vi "VibratomeGUI.vi"(8 "Error Out":errorcluster, 11 "Remote?":bool) -> ()   [LabVIEW 2018]
uses:
  Hardware Mfg/Thorlabs Translation Stages/Controls/Translation Stage Cluster.ctl
  Controls/Translation Stage Types.ctl
  Controls/Translation Stage Quick Status.ctl
  Controls/Translation Stage Quick Controls.ctl
  Controls/QueueNames.ctl
  Controls/Queue Manager Actions.ctl
  Controls/MessagePacket.ctl
  <vilib>/Utility/miscctls.llb/LVPointTypeDef.ctl
  Hardware Mfg/Thorlabs Translation Stages/Controls/Motion Translation Module Control.ctl
  Controls/Set Get Controls.ctl
  Controls/FGV Actions.ctl
panel:
  in  "Z STEP MOTION":enum16{"Fine", "Course", "Extra Course"}(ring)
  in  "Stop Button":bool
  in  "Slice":bool
  in  "Vibratome Controls":T1
  out "Message":string
  in  "Z Ctrl":T2
  out "Z Status":T3
  in  "Y Ctrl":T2
  out "Y Status":T3
  in  "X Ctrl":T2
  out "X Status":T3
  in  "XY STEP MOTION":enum16{"Fine", "Course", "Extra Course"}(ring)
  out "Cluster":cluster{"X":T4, "Y":T4, "Z":T4}
  in  "Exit":bool
  out "Processor Error Out":errorcluster
  out "GUI Error Out":errorcluster
  # "Vibratome Controls"
  # "Z Axis"
  # "Y Axis"
  # "X Axis"
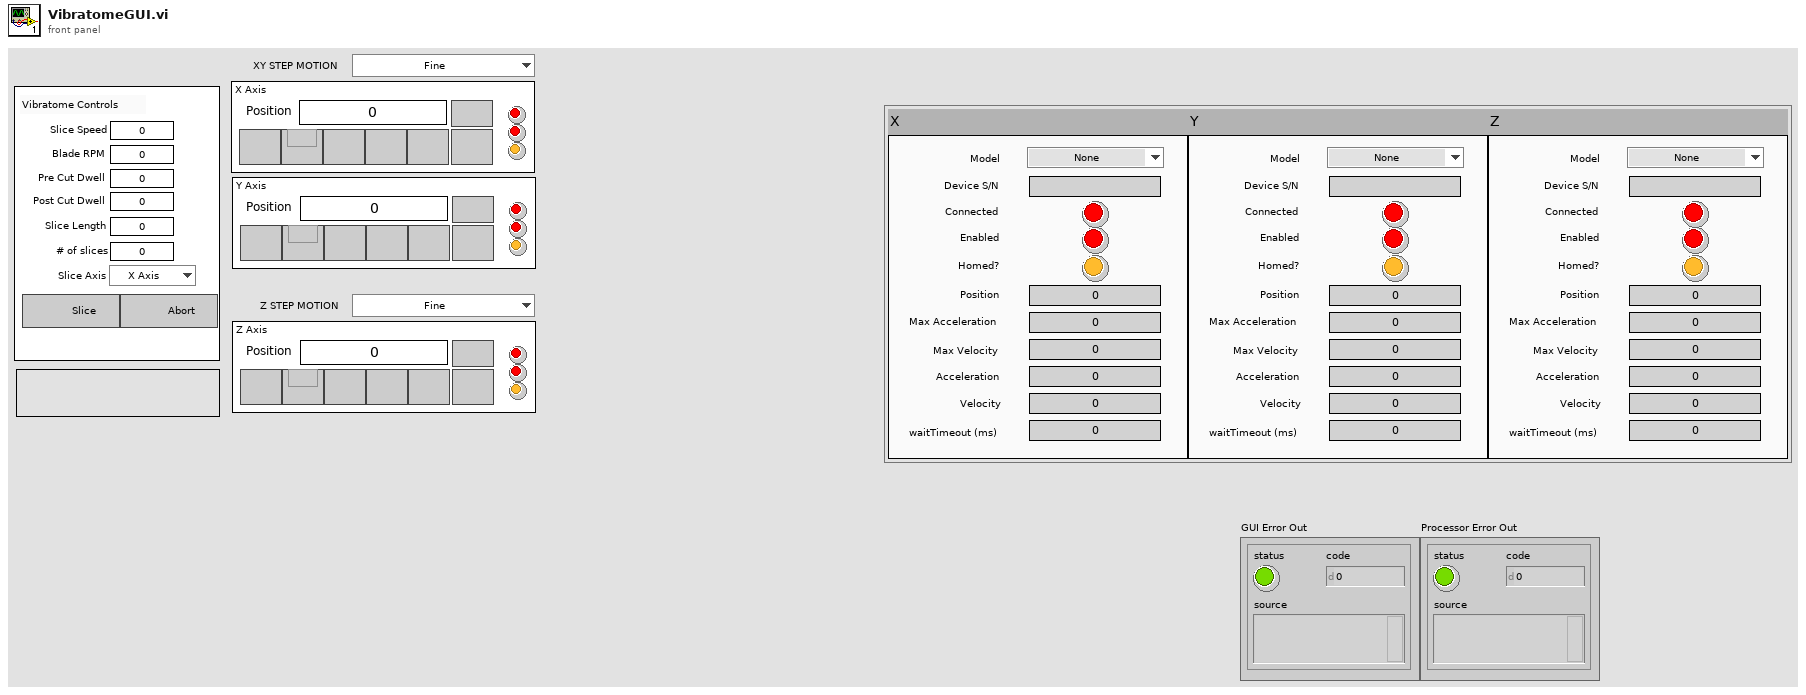
[diagram p1: front panel]
types:
  T1 = cluster{"Pre Cut Dwell":dbl, "Blade RPM":u16, "Slice Speed":dbl, "Post Cut Dwell":dbl, "Slice Length":dbl, "# of slices":dbl, "Slice Axis":enum16{"X Axis", "Y Axis", "Z Axis"}}
  T2 = typedef "Translation Stage Quick Controls.ctl" = cluster{"Position":dbl, "Next Button":bool, "Last Button":bool, "Previous Button":bool, "First Button":bool, "Home Button":bool, "Go":bool, "Settings Button":bool}
  T3 = typedef "Translation Stage Quick Status.ctl" = cluster{"Is.Enabled?":bool, "Is.Connected?":bool, "Is.Homed?":bool}
  T4 = typedef "Translation Stage Cluster.ctl" = cluster{"Position":dbl, "Is.Enabled?":bool, "Is.Connected?":bool, "Device SN":string, "AccelerationMaximum":dbl, "VelocityMaximum":dbl, "Acceleration":dbl, "Velocity":dbl, "waitTimeout (ms)":i32, "Model":T5, "Is.Homed?":bool}
  T5 = typedef "Translation Stage Types.ctl" = enum16{"None", "Thorlabs LTS", "Thorlabs MLJ"}
  T6 = typedef "MessagePacket.ctl" = cluster{"Message":string, "Parameter":variant}
  T7 = typedef "Queue Manager Actions.ctl" = enum16{"Init", "Enqueue", "Enqueue All", "Preview Queue", "Dequeue", "Get Status", "Flush Queue", "Flush All Queues", "Release All Queues", "Release Queue", "Enqueue at Opposite End"}
  T8 = typedef "QueueNames.ctl" = enum16{"Main GUI", "Main Scan Processor", "Main Processing", "Main Saving", "Main Display", "Main Table Stage GUI", "Main Table Stage Proc.", "Scan Engine", "Vibratome GUI", "Vibratome Processor", "Slice Engine"}
  T9 = enum32{"Invalid", "Default", "Floating", "Floating/Auto-Hide", "Modal"}
  T10 = enum32{"Invalid", "Standard", "Closed", "Hidden", "Minimized", "Maximized"}
  T11 = typedef "LVPointTypeDef.ctl" = cluster{"Horizontal":i16, "Vertical":i16}
  T12 = enum16{"Set Configuration", "Get Configuration", "Enable Motor", "Disable Motor", "Get Status", "Open Session", "Close Session", "Set Limits", "Get Limits"}
  T13 = typedef "FGV Actions.ctl" = enum16{"Init", "Set", "Get", "Clear"}
  T14 = typedef "Set Get Controls.ctl" = enum16{"Set", "Get"}
  T15 = typedef "Motion Translation Module Control.ctl" = enum16{"Init", "Home", "Status", "Velocity/Accel", "Position", "Jog", "Stop", "Uninit", "Enable", "Disable"}
  T16 = typedef "Translation Stage Parameters.ctl" = cluster{"X Stage":T4, "Y Stage":T4, "Z Stage":T4}
  T17 = typedef "System Parameters.ctl" = cluster{"Optical Parameters":T18, "Vibratome":T19, "Table Stages":T16, "Imaging Parameter":T20, "Galvo HW Parameters":cluster{"Analog Out Channel":tag, "Min Voltage":dbl, "Max Voltage":dbl, "Pixel Clock Source":tag, "Sample Rate":dbl, "Line Clock Out Ch":tag}, "Alazar parameters":T22, "Mosaic Paramter":cluster{"X Axis":cluster{"Start [mm]":dbl, "Steps [pts]":dbl, "End [mm]":dbl}, "Y Axis":cluster{"Start [mm]":dbl, "Steps [pts]":dbl, "End [mm]":dbl}, "Scan Pattern":enum16{"Uni-directional", "Bi-Directional", "Spiral Out", "Spiral In"}, "Overlap Options":cluster{"Overlap Type":enum16{"No Overlap", "X Only", "Y Only", "X and Y"}, "Percent Overlap":u8, "Justify":enum16{"Start", "Center", "End"}}}, "Manual Controls":T29, "Vibratome Axis":T32}
  T18 = typedef "Optical Parameters.ctl" = cluster{"Obj. Focal Length [mm]":dbl, "Scan Lens EFL[mm]":dbl, "Tube Lens EFL[mm]":dbl, "Galvo V Range (+/-)":dbl, "Galvo Max Half Angle [Deg]":dbl, "Max Galvo Range[%]":dbl}
  T19 = typedef "Vibratome Parameters.ctl" = cluster{"Z Bottom [mm]":dbl, "Pre Cut Dwell [s]":dbl, "Blade Frequency [RPM]":u16, "Slice Speed [mm/s]":dbl, "Post Cut Dwell [s]":dbl, "Ramp Time [s]":dbl, "Start X [mm]":dbl, "Start Y [mm]":dbl, "Slice Length [mm]":dbl, "Slice Axis":enum16{"X Axis", "Y Axis", "Z Axis"}, "Controller VISA Ref":refnum<visa-resource-name>}
  T20 = typedef "Imaging Parameters.ctl" = cluster{"Raster Scan Direction":T21, "Pixel Dwell Time [Clock Cycles]":u16, "Flyback Time [Clock Cycles]":u16, "XY Center [um]":cluster{"X":dbl, "Y":dbl}, "Pixel Step Size [um]":dbl, "XY Image Size":enum16{"32 x 32", "64 x 64", "128 x 128", "256 x 256", "512 x 512", "1024 x 1024", "2048 x 2048"}, "Custom":bool, "Custom Size":cluster{"X":u16, "Y":u16}, "Line Averages":u8}
  T21 = typedef "Scan Direction.ctl" = enum16{"Uni Directional", "Bi Directional", "None"}
  T22 = typedef "Alazar parameters.ctl" = cluster{"Trigger Settings":cluster{"General Trigger Settings":T23, "Trigger Engine 1":T24, "Trigger Engine 2":T24}, "Device ID":T25, "Ch A Input Control":T26, "Ch B Input Control":T26, "Acq Settings":T27, "Capture Clock":T28}
  T23 = typedef "General Trigger Settings.ctl" = cluster{"Trigger Operation":u32, "Coupling ID":u32, "Range ID":u32, "Delay":u32, "Timeout Ticks":u32, "Mode":u32, "Parameter":u32}
  T24 = typedef "Trigger Engine Controls.ctl" = cluster{"Trigger Engine":u32, "Source":u32, "Slope":u32, "Level":u32}
  T25 = typedef "Alazar Device ID.ctl" = cluster{"System ID":u32, "Board ID":u32}
  T26 = typedef "Channel Input Controls.ctl" = cluster{"Channel":u8, "Coupling":u32, "Range":u32, "Impedance":u32}
  T27 = typedef "Alazar Acquisition Settings.ctl" = cluster{"Record Length":u32, "Offset":u32, "Records Per Buffer":u32, "Records Count (Records/Acq)":u32, "Window Type":u32, "Footer":u32, "Samples per record":u32, "Output Format":u32}
  T28 = typedef "Clock Controls.ctl" = cluster{"Sample Rate":u32, "Decimation":u32, "Source":u32, "Edge":u32}
  T29 = typedef "Manual Controls.ctl" = cluster{"Z0":dbl, "Z0 image":dbl, "stripped path":path, "Save parameters":T30, "Center Galvos":bool, "Acquisition mode":T31, "PSOCT Channel":u32, "Save":bool, "AIP rotation angle":dbl, "Scan Parameters":cluster{"# Scan":cluster{"#Ascan":i32, "#Bscan":i32}, "# Rpt":cluster{"#ARpt":i32, "#BRpt":i32}, "Aline Rate":u16, "# Extra":cluster{"# ARpt_extra":i32, "#Brtn_extra":i32}}, "ROI Parameters":cluster{"ROI (mm)":cluster{"X (mm)":dbl, "Y (mm)":dbl}, "Shift (mm)":cluster{"Xshift (mm)":sgl, "Yshift (mm)":sgl}}, "Objective":u16}
  T30 = typedef "FFT parameters.ctl" = cluster{"start pixel":i32, "#pixels to save":i32}
  T31 = typedef "FFT mode.ctl" = enum16{"ThorOCT B line", "ThorOCT Spectral", "ThorOCT FFT", "Alazar B line", "Alazar FFT", "GPU FFT", "Alazar Spectral"}
  T32 = typedef "Vibratome Param.ctl" = cluster{"Start [mm](Next cut height)":dbl, "thick slice[um]":dbl, "#repitition":u16, "thin slice[um]":dbl, "#thin slices":u16}
  T33 = cluster{"Z Bottom [mm]":dbl, "Pre Cut Dwell [s]":dbl, "Blade Frequency [RPM]":u16, "Slice Speed [mm/s]":dbl, "Post Cut Dwell [s]":dbl, "Ramp Time [s]":dbl, "Start X [mm]":dbl, "Start Y [mm]":dbl, "Slice Length [mm]":dbl, "Slice Axis":enum16{"X Axis", "Y Axis", "Z Axis"}, "Controller VISA Ref":refnum<visa-resource-name>}
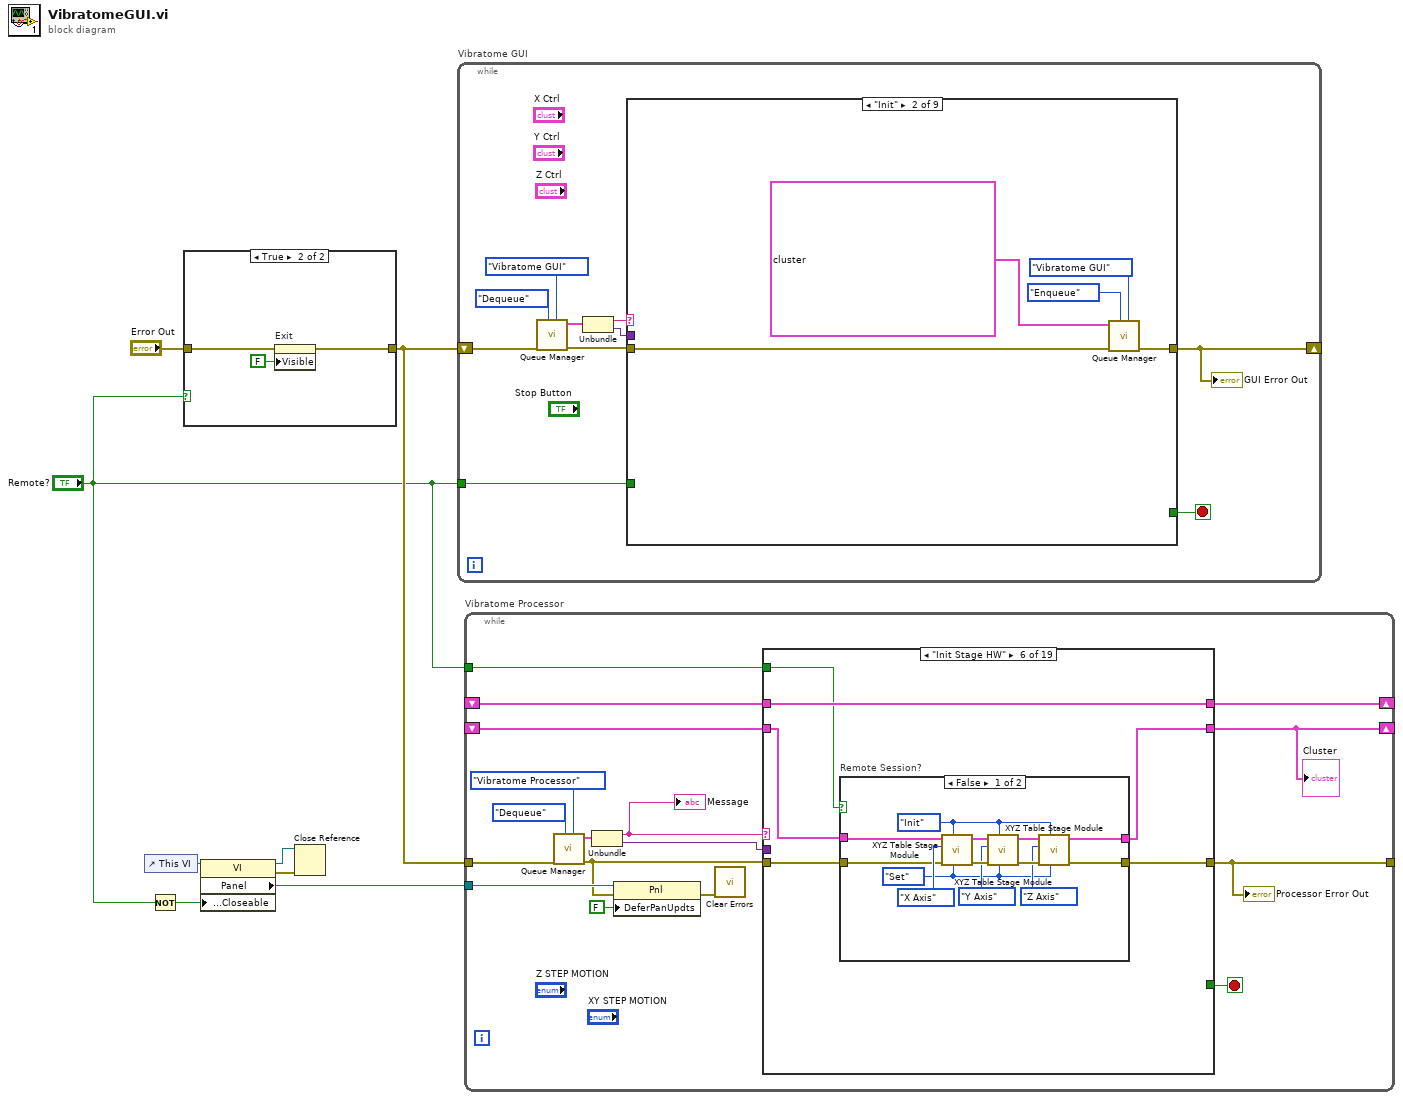
[diagram p0: block diagram]
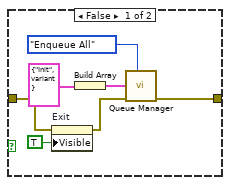
[diagram p2: hidden frame]
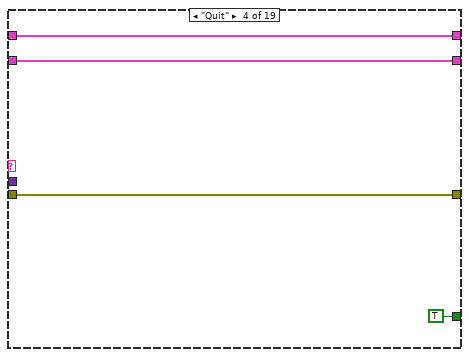
[diagram p6: hidden frame]
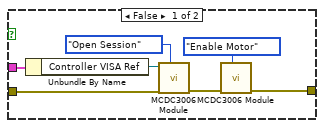
[diagram p10: hidden frame]
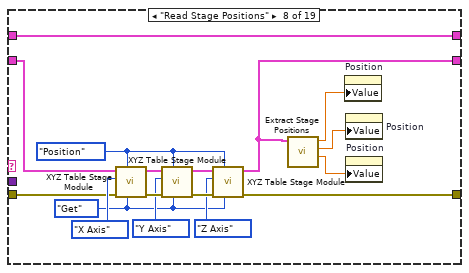
[diagram p11: hidden frame]
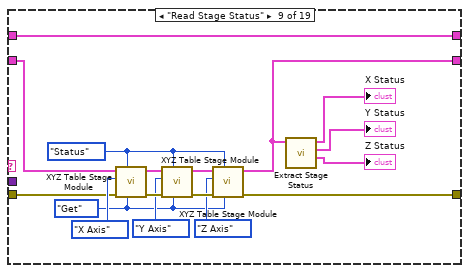
[diagram p12: hidden frame]
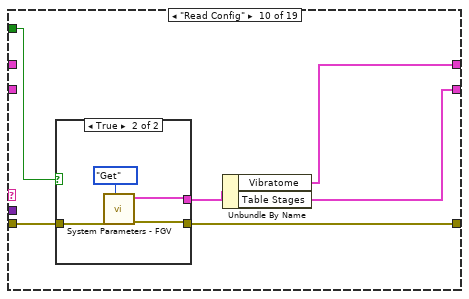
[diagram p13: hidden frame]
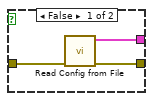
[diagram p14: hidden frame]
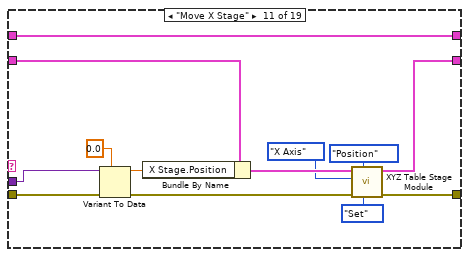
[diagram p15: hidden frame]
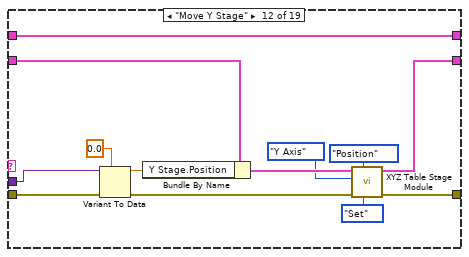
[diagram p16: hidden frame]
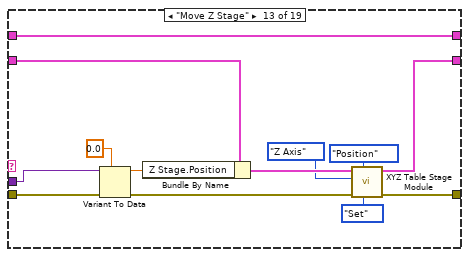
[diagram p17: hidden frame]
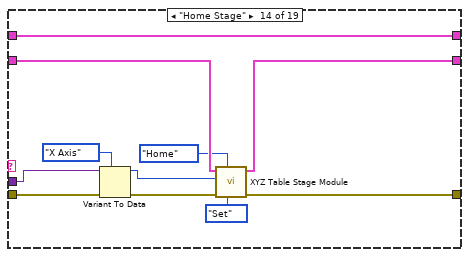
[diagram p18: hidden frame]
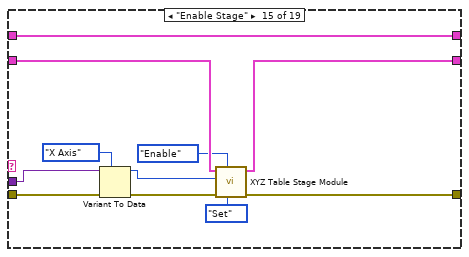
[diagram p19: hidden frame]
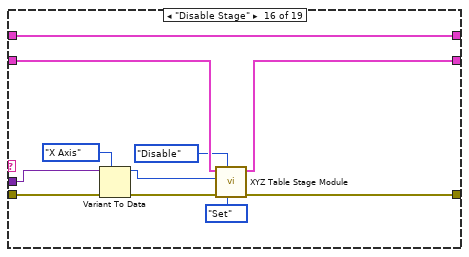
[diagram p20: hidden frame]
diagram:
  n1 = control-ref of="This VI"() -> (w7:refnum<vi>)
  n2 = Not(x="Remote?") -> (.not. x?=w1:bool)
  n3 = case shown="True" "Remote?" {
    tunnel: [w12 w17] -> w8
    tunnel: "Error Out" -> [w10 w18]
    frame False {
      n4 = property on="Exit" class="Bool"(error in=w10, "Visible"=TRUE) -> (error out=w9:errorcluster)  [unwired: 1 in, 1 out]
      n5 = Build Array(T6 {"Message"="Init", "Parameter"=variant} ("Message Packet [In]")) -> (w13:T6[])
      n6 = call "Queue Manager.vi"("Action"=Queue_Manager_Actions."Enqueue All", "Error In"=w9, "Message Packet Array"=w13) -> ("Error Out"=w12:errorcluster)  [unwired: 4 in, 4 out]
    }
    frame True {
      n7 = property on="Exit" class="Bool"(error in=w18, "Visible"=FALSE) -> (error out=w17:errorcluster)  [unwired: 1 in, 1 out]
    }
  }
  n8 = property class="VI"(reference=w7, "Front Panel.Closeable"=w1) -> (reference out=w5:refnum<vi>, error out=w6:errorcluster, "Panel"=w4:refnum<vi>)  [unwired: 1 in]
  n9 = Close Reference(reference=w5, error in (no error)=w6) -> ()  [unwired: 1 out]
  n10 = while "Vibratome GUI" {
    shift-right: [w28] -> _
    shift-left: w8 -> [w26]
    tunnel: "Remote?" -> [w19]
    stop <- w21 stop-if-true
    n11 = call "Queue Manager.vi"("Queue Name"=QueueNames."Vibratome GUI", "Action"=Queue_Manager_Actions."Dequeue", "Error In"=w26) -> ("Error Out"=w25:errorcluster, "Message Packet [Out]"=w24:T6)  [unwired: 4 in, 3 out]
    n12 = Unbundle(w24) -> ("Message"=w23:string, "Parameter"=w22:variant)
    n13 = case shown="\"Init\"" w23 {
      tunnel: w25 -> [w29 w30 w35 w36 w38 w42 w45 w118 w130]
      tunnel: [w29 w31 w35 w36 w37 w42 w44 w119 w130] -> w28
      tunnel: w22 -> [_ _ _ _ _ _ _ _ _]
      tunnel: [_ _ _ _ _ _ _ _ TRUE] -> w21
      tunnel: w19 -> [_ _ _ _ _ _ w43 w113 _]
      frame "Unknown", Default {
      }
      frame "Init" {
        n14 = call "Queue Manager.vi"("Queue Name"=QueueNames."Vibratome GUI", "Action"=Queue_Manager_Actions."Enqueue", "Error In"=w30, "Message Packet Array"=T6[] [{"Message"="Init Variables", "Parameter"=variant}, {"Message"="Set Front Panel", "Parameter"=variant}, {"Message"="Load User Settings", "Parameter"=variant}, {"Message"="Configure Hardware", "Parameter"=variant}, {"Message"="Wait for Complete", "Parameter"=variant}, {"Message"="Wait for User Input", "Parameter"=variant}]) -> ("Error Out"=w31:errorcluster)  [unwired: 3 in, 4 out]
      }
      frame "Init Variables" {
      }
      frame "Load User Settings" {
      }
      frame "Configure Hardware" {
        n15 = call "Queue Manager.vi"("Queue Name"=QueueNames."Vibratome Processor", "Action"=Queue_Manager_Actions."Enqueue", "Error In"=w38, "Message Packet Array"=T6[] [{"Message"="Read Config", "Parameter"=variant}, {"Message"="Init Stage HW", "Parameter"=variant}, {"Message"="Read Stage Status", "Parameter"=variant}, {"Message"="Read Stage Positions", "Parameter"=variant}, {"Message"="Init Vibratome HW", "Parameter"=variant}, {"Message"="Finished Init", "Parameter"=variant}]) -> ("Error Out"=w37:errorcluster)  [unwired: 3 in, 4 out]
      }
      frame "Wait for Complete" {
      }
      frame "Wait for User Input" {
        n16 = event shown="[1] Panel Close;  Application Instance Close;  \"Exit\": Value Change" {
          selector: _ -> [_ _ _ _ _ _]
          dyn-events: _ -> [_ _ _ _ _ _]
          timeout: _ -> [_ _ _ _ _ _]
          tunnel: w45 -> [w46 w49 w57 w79 w94 w109]
          tunnel: [w46 w48 w62 w66 w81 w96] -> w44
          tunnel: w43 -> [_ w47 _ _ _ _]
          event Timeout {
            n17 = event-data() -> ()  [unwired: 1 in, 3 out]
          }
          event Panel Close; Application Instance Close; "Exit": Value Change {
            n18 = event-data() -> ()  [unwired: 1 in, 3 out]
            n19 = case shown="True" w47 {
              tunnel: w49 -> [w53 w55]
              tunnel: [w52 w55] -> w48
              frame False {
                n20 = Build Array(T6 {"Message"="Exit", "Parameter"=variant} ("Message Packet [In]")) -> (w50:T6[])
                n21 = call "Queue Manager.vi"("Action"=Queue_Manager_Actions."Enqueue All", "Error In"=w53, "Message Packet Array"=w50) -> ("Error Out"=w52:errorcluster)  [unwired: 4 in, 4 out]
              }
              frame True {
              }
            }
          }
          event "Slice": Value Change {
            n22 = event-data() -> ()  [unwired: 1 in, 6 out]
            n23 = Build Array(T6 {"Message"="Wait for User Input", "Parameter"=variant} ("Message Packet [In]")) -> (w60:T6[])
            n24 = call "Queue Manager.vi"("Queue Name"=QueueNames."Vibratome GUI", "Action"=Queue_Manager_Actions."Enqueue", "Error In"=w57, "Message Packet Array"=w60) -> ("Error Out"=w62:errorcluster)  [unwired: 3 in, 4 out]
            n25 = call "Queue Manager.vi"("Queue Name"=QueueNames."Vibratome Processor", "Action"=Queue_Manager_Actions."Enqueue", "Error In"=w57, "Message Packet Array"=T6[] [{"Message"="Slice", "Parameter"=variant}, {"Message"="Finished", "Parameter"=variant}]) -> ()  [unwired: 3 in, 5 out]
          }
          event Value Change {
            n26 = event-data() -> ()  [unwired: 1 in, 1 out]
            n27 = property on="Position" class="DigNum (strict)"(error in=w79) -> (error out=w76:errorcluster, "Value"=w74:dbl)  [unwired: 1 in, 1 out]
            n28 = Bundle By Name(cluster=T6 {"Message"="Move X Stage", "Parameter"=variant} ("Message Packet [In]"), "Parameter"=w74) -> (w73:T6)
            n29 = Build Array(w73, T6 {"Message"="Finished", "Parameter"=variant} ("Message Packet [In]")) -> (w72:T6[])
            n30 = call "Queue Manager.vi"("Queue Name"=QueueNames."Vibratome Processor", "Action"=Queue_Manager_Actions."Enqueue", "Error In"=w76, "Message Packet Array"=w72) -> ("Error Out"=w67:errorcluster)  [unwired: 3 in, 4 out]
            n31 = Build Array(T6 {"Message"="Wait for User Input", "Parameter"=variant} ("Message Packet [In]")) -> (w68:T6[])
            n32 = call "Queue Manager.vi"("Queue Name"=QueueNames."Vibratome GUI", "Action"=Queue_Manager_Actions."Enqueue", "Error In"=w67, "Message Packet Array"=w68) -> ("Error Out"=w66:errorcluster)  [unwired: 3 in, 4 out]
          }
          event Value Change {
            n33 = event-data() -> ()  [unwired: 1 in, 1 out]
            n34 = property on="Position" class="DigNum (strict)"(error in=w94) -> (error out=w91:errorcluster, "Value"=w89:dbl)  [unwired: 1 in, 1 out]
            n35 = Bundle By Name(cluster=T6 {"Message"="Move Y Stage", "Parameter"=variant} ("Message Packet [In]"), "Parameter"=w89) -> (w88:T6)
            n36 = Build Array(w88, T6 {"Message"="Finished", "Parameter"=variant} ("Message Packet [In]")) -> (w87:T6[])
            n37 = call "Queue Manager.vi"("Queue Name"=QueueNames."Vibratome Processor", "Action"=Queue_Manager_Actions."Enqueue", "Error In"=w91, "Message Packet Array"=w87) -> ("Error Out"=w82:errorcluster)  [unwired: 3 in, 4 out]
            n38 = Build Array(T6 {"Message"="Wait for User Input", "Parameter"=variant} ("Message Packet [In]")) -> (w83:T6[])
            n39 = call "Queue Manager.vi"("Queue Name"=QueueNames."Vibratome GUI", "Action"=Queue_Manager_Actions."Enqueue", "Error In"=w82, "Message Packet Array"=w83) -> ("Error Out"=w81:errorcluster)  [unwired: 3 in, 4 out]
          }
          event Value Change {
            n40 = event-data() -> ()  [unwired: 1 in, 1 out]
            n41 = property on="Position" class="DigNum (strict)"(error in=w109) -> (error out=w106:errorcluster, "Value"=w104:dbl)  [unwired: 1 in, 1 out]
            n42 = Bundle By Name(cluster=T6 {"Message"="Move Z Stage", "Parameter"=variant} ("Message Packet [In]"), "Parameter"=w104) -> (w103:T6)
            n43 = Build Array(w103, T6 {"Message"="Finished", "Parameter"=variant} ("Message Packet [In]")) -> (w102:T6[])
            n44 = call "Queue Manager.vi"("Queue Name"=QueueNames."Vibratome Processor", "Action"=Queue_Manager_Actions."Enqueue", "Error In"=w106, "Message Packet Array"=w102) -> ("Error Out"=w97:errorcluster)  [unwired: 3 in, 4 out]
            n45 = Build Array(T6 {"Message"="Wait for User Input", "Parameter"=variant} ("Message Packet [In]")) -> (w98:T6[])
            n46 = call "Queue Manager.vi"("Queue Name"=QueueNames."Vibratome GUI", "Action"=Queue_Manager_Actions."Enqueue", "Error In"=w97, "Message Packet Array"=w98) -> ("Error Out"=w96:errorcluster)  [unwired: 3 in, 4 out]
          }
        }
      }
      frame "Set Front Panel" {
        n47 = Select(t=T10."Hidden" ("Front Panel Window:State"), s=w113, f=T10."Standard" ("Front Panel Window:State")) -> (s? t:f=w114:T10)
        n48 = control-ref of="This VI"() -> (w117:refnum<vi>)
        n49 = Select(t=T9."Default" ("Front Panel Window:Behavior"), s=w113, f=T9."Modal") -> (s? t:f=w110:T9)
        n50 = property class="VI"(reference=w117, error in=w118, "FP.State"=w114, "FP.Behavior"=w110) -> (error out=w121:errorcluster, "Panel"=w124:refnum<vi>)  [unwired: 1 out]
        n51 = property class="Pnl"(reference=w124, error in=w121) -> (error out=w122:errorcluster, "Panes[]"=w123:refnum<vi>[])  [unwired: 1 out]
        n52 = for {
          tunnel: w123 -> [w128] mode=indexing
          tunnel: w122 -> [w126]
          tunnel: [w125] -> w120 mode=indexing
          n53 = property class="Pane"(reference=w128, error in=w126, "Origin"=T11 {"Horizontal"=0, "Vertical"=0}) -> (error out=w125:errorcluster)  [unwired: 1 out]
        }
        n54 = Merge Errors(w120) -> (w119:errorcluster)
      }
      frame "Exit" {
      }
    }
    "GUI Error Out" <- w28
  }
  n55 = while "Vibratome Processor" {
    tunnel: w8 -> [w145]
    tunnel: [w147] -> _
    shift-right: [w136] -> _
    shift-left: _ -> [w139]
    shift-right: [w138] -> _
    shift-left: _ -> [w137]
    tunnel: w4 -> [w135]
    tunnel: "Remote?" -> [w131]
    stop <- w141 stop-if-true
    n56 = call "Queue Manager.vi"("Queue Name"=QueueNames."Vibratome Processor", "Action"=Queue_Manager_Actions."Dequeue", "Error In"=w145) -> ("Error Out"=w133:errorcluster, "Message Packet [Out]"=w144:T6)  [unwired: 4 in, 3 out]
    n57 = Unbundle(w144) -> ("Message"=w143:string, "Parameter"=w142:variant)
    "Message" <- w143
    n58 = property class="Pnl"(reference=w135, error in=w133, "DeferPanUpdts"=FALSE ("Defer Panel Updates")) -> (error out=w132:errorcluster)  [unwired: 1 out]
    n59 = call <vilib>:"Clear Errors.vi"("error in (no error)"=w132) -> ()  [unwired: 5 in, 2 out]
    n60 = case shown="\"Init Stage HW\"" w143 {
      tunnel: w133 -> [w150 w153 w154 w158 w161 w166 w186 w202 w219 w235 w255 w268 w281 w292 w303 w314 w319 w325 w345]
      tunnel: [w150 w153 w154 w158 w161 w167 w184 w210 w227 w233 w254 w267 w280 w291 w302 w313 w318 w324 w329] -> w147
      tunnel: w142 -> [_ _ _ _ _ _ _ _ _ _ w252 w265 w278 w289 w300 w311 _ _ _]
      tunnel: [_ _ _ TRUE _ _ _ _ _ _ _ _ _ _ _ _ _ _ _] -> w141
      tunnel: [w149 w152 w156 w160 _ w163 w187 w196 w217 w234 w251 w264 w277 w285 w296 w307 w316 w326 w338] -> w136
      tunnel: w139 -> [w149 w152 w156 w160 _ w165 w187 w201 w218 _ w247 w260 w273 w286 w297 w308 w316 w326 w341]
      tunnel: [w148 w151 w155 w159 _ w164 w185 w200 w213 w232 w243 w256 w269 w282 w293 w304 w320 w327 w332] -> w138
      tunnel: w137 -> [w148 w151 w155 w159 _ w164 w185 w200 w213 _ w243 w256 w269 w282 w293 w304 w320 w327 w332]
      tunnel: w131 -> [_ _ _ _ _ w162 w183 _ _ w230 _ _ _ _ _ _ _ _ _]
      frame "Unknown", Default {
      }
      frame "Finished Init" {
      }
      frame "Finished" {
      }
      frame "Quit" {
      }
      frame "Init" {
      }
      frame "Init Stage HW" {
        n61 = case "Remote Session?" shown="False" w162 {
          tunnel: [w178 w181] -> w167
          tunnel: w166 -> [w170 w181]
          tunnel: w165 -> [w169 w182]
          tunnel: [w168 w182] -> w163
          frame False {
            w171 = Set_Get_Controls."Set" ("Set/Get")
            w177 = Motion_Translation_Module_Control."Init" ("Action")
            n62 = call "XYZ Table Stage Module.vi"("Set/Get"=w171, "Action"=w177, "Error In"=w170, "Axis"=enum16{"X Axis", "Y Axis", "Z Axis"}."X Axis", "Table Stages"=w169) -> ("Error Out"=w180:errorcluster, "Table Stages [out]"=w176:T16)  [unwired: 5 in]
            n63 = call "XYZ Table Stage Module.vi"("Set/Get"=w171, "Action"=w177, "Error In"=w180, "Axis"=enum16{"X Axis", "Y Axis", "Z Axis"}."Y Axis", "Table Stages"=w176) -> ("Error Out"=w179:errorcluster, "Table Stages [out]"=w175:T16)  [unwired: 5 in]
            n64 = call "XYZ Table Stage Module.vi"("Set/Get"=w171, "Action"=w177, "Error In"=w179, "Axis"=enum16{"X Axis", "Y Axis", "Z Axis"}."Z Axis", "Table Stages"=w175) -> ("Error Out"=w178:errorcluster, "Table Stages [out]"=w168:T16)  [unwired: 5 in]
          }
          frame True {
          }
        }
      }
      frame "Init Vibratome HW" {
        n65 = case "Remote Session?" shown="True" w183 {
          tunnel: w186 -> [w193 w195]
          tunnel: w185 -> [w191 _]
          tunnel: [w189 w195] -> w184
          frame False {
            n66 = Unbundle By Name(w191) -> ("Controller VISA Ref"=w190:refnum<visa-resource-name>)
            n67 = call "MCDC3006 Module.vi"("Actions"=T12."Open Session", "Error In"=w193, "VISA resource name"=w190) -> ("Error Out"=w192:errorcluster)  [unwired: 4 in, 4 out]
            n68 = call "MCDC3006 Module.vi"("Actions"=T12."Enable Motor", "Error In"=w192) -> ("Error Out"=w189:errorcluster)  [unwired: 5 in, 4 out]
          }
          frame True {
          }
        }
      }
      frame "Read Stage Positions" {
        w203 = Set_Get_Controls."Get" ("Set/Get")
        w209 = Motion_Translation_Module_Control."Position" ("Action")
        n69 = call "XYZ Table Stage Module.vi"("Set/Get"=w203, "Action"=w209, "Error In"=w202, "Axis"=enum16{"X Axis", "Y Axis", "Z Axis"}."X Axis", "Table Stages"=w201) -> ("Error Out"=w212:errorcluster, "Table Stages [out]"=w208:T16)  [unwired: 5 in]
        n70 = call "XYZ Table Stage Module.vi"("Set/Get"=w203, "Action"=w209, "Error In"=w212, "Axis"=enum16{"X Axis", "Y Axis", "Z Axis"}."Y Axis", "Table Stages"=w208) -> ("Error Out"=w211:errorcluster, "Table Stages [out]"=w207:T16)  [unwired: 5 in]
        n71 = call "XYZ Table Stage Module.vi"("Set/Get"=w203, "Action"=w209, "Error In"=w211, "Axis"=enum16{"X Axis", "Y Axis", "Z Axis"}."Z Axis", "Table Stages"=w207) -> ("Error Out"=w210:errorcluster, "Table Stages [out]"=w196:T16)  [unwired: 5 in]
        n72 = call "Extract Stage Positions.vi"("Table Stages"=w196) -> ("Z Stage.Position"=w197:dbl, "Y Stage.Position"=w198:dbl, "X Stage.Position"=w199:dbl)  [unwired: 8 in]
        n73 = property on="Position" class="DigNum (strict)"("Value"=w199) -> ()  [unwired: 2 in, 2 out]
        n74 = property on="Position" class="DigNum (strict)"("Value"=w198) -> ()  [unwired: 2 in, 2 out]
        n75 = property on="Position" class="DigNum (strict)"("Value"=w197) -> ()  [unwired: 2 in, 2 out]
      }
      frame "Read Stage Status" {
        w220 = Set_Get_Controls."Get" ("Set/Get")
        w226 = Motion_Translation_Module_Control."Status" ("Action")
        n76 = call "XYZ Table Stage Module.vi"("Set/Get"=w220, "Action"=w226, "Error In"=w219, "Axis"=enum16{"X Axis", "Y Axis", "Z Axis"}."X Axis", "Table Stages"=w218) -> ("Error Out"=w229:errorcluster, "Table Stages [out]"=w225:T16)  [unwired: 5 in]
        n77 = call "XYZ Table Stage Module.vi"("Set/Get"=w220, "Action"=w226, "Error In"=w229, "Axis"=enum16{"X Axis", "Y Axis", "Z Axis"}."Y Axis", "Table Stages"=w225) -> ("Error Out"=w228:errorcluster, "Table Stages [out]"=w224:T16)  [unwired: 5 in]
        n78 = call "XYZ Table Stage Module.vi"("Set/Get"=w220, "Action"=w226, "Error In"=w228, "Axis"=enum16{"X Axis", "Y Axis", "Z Axis"}."Z Axis", "Table Stages"=w224) -> ("Error Out"=w227:errorcluster, "Table Stages [out]"=w217:T16)  [unwired: 5 in]
        n79 = call "Extract Stage Status.vi"("Table Stages"=w217) -> ("Z Stage"=→"Z Status":T3, "Y Stage"=→"Y Status":T3, "X Stage"=→"X Status":T3)  [unwired: 8 in]
      }
      frame "Read Config" {
        n80 = case shown="True" w230 {
          tunnel: w235 -> [w238 w241]
          tunnel: [w237 w240] -> w233
          tunnel: [w236 w239] -> w231
          frame False {
            n81 = call "Read Config from File.vi"("error in (no error)"=w238) -> ("error out"=w237:errorcluster, "System Parameters"=w236:T17)  [unwired: 9 in]
          }
          frame True {
            n82 = call "System Parameters - FGV.vi"("Actions"=FGV_Actions."Get", "Error In"=w241) -> ("Error Out"=w240:errorcluster, "System Parameters [Out]"=w239:T17)  [unwired: 8 in]
          }
        }
        n83 = Unbundle By Name(w231) -> ("Vibratome"=w232:T19, "Table Stages"=w234:T16)
      }
      frame "Move X Stage" {
        n84 = Variant To Data(error in=w255, type=0.0 ("Value"), Variant=w252) -> (data=w246:dbl, error out=w253:errorcluster)
        n85 = Bundle By Name(cluster=w247, "X Stage.Position"=w246) -> (w245:T16)
        n86 = call "XYZ Table Stage Module.vi"("Set/Get"=Set_Get_Controls."Set", "Action"=Motion_Translation_Module_Control."Position", "Error In"=w253, "Axis"=enum16{"X Axis", "Y Axis", "Z Axis"}."X Axis", "Table Stages"=w245) -> ("Error Out"=w254:errorcluster, "Table Stages [out]"=w251:T16)  [unwired: 5 in]
      }
      frame "Move Y Stage" {
        n87 = Variant To Data(error in=w268, type=0.0 ("Value"), Variant=w265) -> (data=w259:dbl, error out=w266:errorcluster)
        n88 = Bundle By Name(cluster=w260, "Y Stage.Position"=w259) -> (w258:T16)
        n89 = call "XYZ Table Stage Module.vi"("Set/Get"=Set_Get_Controls."Set", "Action"=Motion_Translation_Module_Control."Position", "Error In"=w266, "Axis"=enum16{"X Axis", "Y Axis", "Z Axis"}."Y Axis", "Table Stages"=w258) -> ("Error Out"=w267:errorcluster, "Table Stages [out]"=w264:T16)  [unwired: 5 in]
      }
      frame "Move Z Stage" {
        n90 = Variant To Data(error in=w281, type=0.0 ("Value"), Variant=w278) -> (data=w272:dbl, error out=w279:errorcluster)
        n91 = Bundle By Name(cluster=w273, "Z Stage.Position"=w272) -> (w271:T16)
        n92 = call "XYZ Table Stage Module.vi"("Set/Get"=Set_Get_Controls."Set", "Action"=Motion_Translation_Module_Control."Position", "Error In"=w279, "Axis"=enum16{"X Axis", "Y Axis", "Z Axis"}."Z Axis", "Table Stages"=w271) -> ("Error Out"=w280:errorcluster, "Table Stages [out]"=w277:T16)  [unwired: 5 in]
      }
      frame "Home Stage" {
        n93 = Variant To Data(error in=w292, type=enum16{"X Axis", "Y Axis", "Z Axis"}."X Axis" ("Axis"), Variant=w289) -> (data=w287:enum16{"X Axis", "Y Axis", "Z Axis"}, error out=w290:errorcluster)
        n94 = call "XYZ Table Stage Module.vi"("Set/Get"=Set_Get_Controls."Set", "Action"=Motion_Translation_Module_Control."Home", "Error In"=w290, "Axis"=w287, "Table Stages"=w286) -> ("Error Out"=w291:errorcluster, "Table Stages [out]"=w285:T16)  [unwired: 5 in]
      }
      frame "Enable Stage" {
        n95 = Variant To Data(error in=w303, type=enum16{"X Axis", "Y Axis", "Z Axis"}."X Axis" ("Axis"), Variant=w300) -> (data=w298:enum16{"X Axis", "Y Axis", "Z Axis"}, error out=w301:errorcluster)
        n96 = call "XYZ Table Stage Module.vi"("Set/Get"=Set_Get_Controls."Set", "Action"=Motion_Translation_Module_Control."Enable", "Error In"=w301, "Axis"=w298, "Table Stages"=w297) -> ("Error Out"=w302:errorcluster, "Table Stages [out]"=w296:T16)  [unwired: 5 in]
      }
      frame "Disable Stage" {
        n97 = Variant To Data(error in=w314, type=enum16{"X Axis", "Y Axis", "Z Axis"}."X Axis" ("Axis"), Variant=w311) -> (data=w309:enum16{"X Axis", "Y Axis", "Z Axis"}, error out=w312:errorcluster)
        n98 = call "XYZ Table Stage Module.vi"("Set/Get"=Set_Get_Controls."Set", "Action"=Motion_Translation_Module_Control."Disable", "Error In"=w312, "Axis"=w309, "Table Stages"=w308) -> ("Error Out"=w313:errorcluster, "Table Stages [out]"=w307:T16)  [unwired: 5 in]
      }
      frame "Slice" {
        n99 = call "Extract Vibratome.vi"("Vibratome Controls"="Vibratome Controls", "Vibratome"=w320) -> ("Vibratome Out"=w317:T33)  [unwired: 9 in]
        n100 = call "Slice Module.vi"("Error In"=w319, "Table Stages"=w316, "Vibratome"=w317) -> ("Error Out"=w318:errorcluster)  [unwired: 6 in, 2 out]
      }
      frame "Exit" {
        n101 = call "Queue Manager.vi"("Queue Name"=QueueNames."Vibratome Processor", "Action"=Queue_Manager_Actions."Enqueue", "Error In"=w325, "Message Packet Array"=T6[] [{"Message"="Uninit", "Parameter"=variant}, {"Message"="Quit", "Parameter"=variant}]) -> ("Error Out"=w324:errorcluster)  [unwired: 3 in, 4 out]
      }
      frame "Uninit" {
        w333 = Set_Get_Controls."Set" ("Set/Get")
        w337 = Motion_Translation_Module_Control."Uninit" ("Action")
        n102 = call "XYZ Table Stage Module.vi"("Set/Get"=w333, "Action"=w337, "Error In"=w345, "Axis"=enum16{"X Axis", "Y Axis", "Z Axis"}."X Axis", "Table Stages"=w341) -> ("Error Out"=w343:errorcluster, "Table Stages [out]"=w340:T16)  [unwired: 5 in]
        n103 = call "XYZ Table Stage Module.vi"("Set/Get"=w333, "Action"=w337, "Error In"=w343, "Axis"=enum16{"X Axis", "Y Axis", "Z Axis"}."Y Axis", "Table Stages"=w340) -> ("Error Out"=w344:errorcluster, "Table Stages [out]"=w339:T16)  [unwired: 5 in]
        n104 = call "XYZ Table Stage Module.vi"("Set/Get"=w333, "Action"=w337, "Error In"=w344, "Axis"=enum16{"X Axis", "Y Axis", "Z Axis"}."Z Axis", "Table Stages"=w339) -> ("Error Out"=w342:errorcluster, "Table Stages [out]"=w338:T16)  [unwired: 5 in]
        n105 = call "MCDC3006 Module.vi"("Actions"=T12."Disable Motor", "Error In"=w342) -> ("Error Out"=w331:errorcluster)  [unwired: 5 in, 4 out]
        n106 = call "MCDC3006 Module.vi"("Actions"=T12."Close Session", "Error In"=w331) -> ("Error Out"=w329:errorcluster)  [unwired: 5 in, 4 out]
      }
    }
    "Processor Error Out" <- w147
    "Cluster" <- w136
  }
